vi "TEST Get Wind Speeds.vi"() -> ()   [LabVIEW 2009]
doc: "This is is part of the test process for the Wind Turbine SEQ class. It works in conjunction with the TEST Set Wind Speeds.vi\n\nAAL 9/09"
panel:
  in  "Exit":bool
  out "Turbines":dbl[](array[numeric])
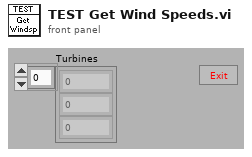
[diagram p1: front panel]
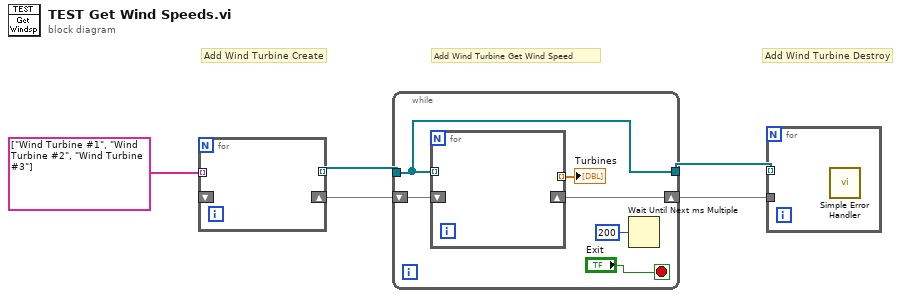
[diagram p0: block diagram]
diagram:
  # "Add Wind Turbine Destroy"
  # "Add Wind Turbine Get Wind Speed"
  # "Add Wind Turbine Create"
  n1 = for {
    tunnel: string[] ["Wind Turbine #1", "Wind Turbine #2", "Wind Turbine #3"] -> [w8] mode=indexing
    tunnel: [w9] -> w4 mode=indexing
    shift-right: [w7] -> w2
    shift-left: _ -> [w6]
  }
  n2 = while {
    tunnel: w4 -> [w14]
    tunnel: [w14] -> w3
    shift-right: [w10] -> w1
    shift-left: w2 -> [w11]
    stop <- "Exit" stop-if-true
    n3 = for {
      tunnel: w14 -> [_] mode=indexing
      tunnel: [w17] -> w15 mode=indexing
      shift-right: [w16] -> w10
      shift-left: w11 -> [_]
    }
    "Turbines" <- w15
    n4 = Wait Until Next ms Multiple(millisecond multiple=u32 200) -> ()  [unwired: 1 out]
  }
  n5 = for {
    tunnel: w3 -> [_] mode=indexing
    tunnel: w1 -> [_]
    n6 = call <vilib>:"Simple Error Handler.vi"() -> ()  [unwired: 2 in, 8 out]
  }
